vi "Indentation.vi"(1 "Index":u32) -> (0 "Indentation":string)   [LabVIEW 2015, in "YAML Parser.lvlib"]
uses:
  YAML Parser.lvlib
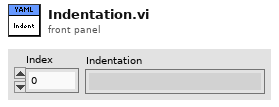
[diagram p1: front panel]
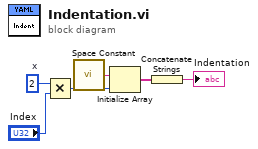
[diagram p0: block diagram]
diagram:
  w3 = u32 2  # x
  n1 = Multiply(x=w3, y="Index") -> (x*y=w4:u32)
  n2 = call <vilib>:"Space Constant.vi"() -> ("String"=w6:string)
  n3 = Initialize Array(w6, w4) -> (w5:string[])
  n4 = Concatenate Strings(w5) -> (→"Indentation":string)
